vi "Eliminated.vi"(6 "Column":i32, 8 "Row":i32, 9 "Killer":i32, 10 "Team":i32, 11 "AntFarm_MB in":refnum<class "AntFarm_MB.lvclass">) -> (3 "AntFarm_MB out":refnum<class "AntFarm_MB.lvclass">)   [LabVIEW 2017, in "AntFarm_MB.lvclass"]
uses:
  AntFarm_MB.lvclass
  TypeDefs/Cluster_Square Data.ctl
  TypeDefs/ENUM_Position ID.ctl
  Type Defs/Direction Enum.ctl
  Type Defs/Action Enum.ctl
  AntFarm_MB.lvclass/AntFarm_MB.ctl
  Square/Square.lvclass
  Type Defs/SB Type Defs.lvlib
panel:
  out "Data":T1
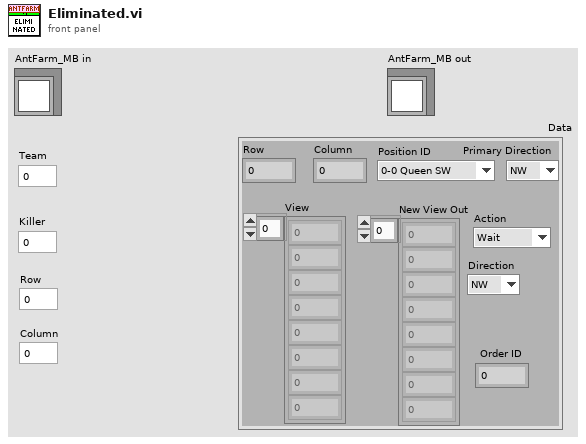
[diagram p1: front panel]
types:
  T1 = typedef "Cluster_Square Data.ctl" = cluster{"Row":i32, "Column":i32, "Position ID":T2, "Primary Direction":T3, "Action":T4, "Direction":T3, "View":i32[], "New View Out":i32[], "Order ID":i32}
  T2 = typedef "ENUM_Position ID.ctl" = enum16{"0-0 Queen SW", "0-1 Path E", "0-2 Queen NW", "0-3 Path W", "1-0 Path S", "1-1 Larva SW", "1-2 Path N", "1-3 Larva NW", "2-0 Queen SE", "2-1 Path W", "2-2 Queen NE", "2-3 Path E", "3-0 Path N", "3-1 Larva SE", "3-2 Path S", "3-3 Larva NE"}
  T3 = typedef "SB Type Defs.lvlib/Direction Enum.ctl" = enum16{"NW", "N", "NE", "E", "SE", "S", "SW", "W"}
  T4 = typedef "SB Type Defs.lvlib/Action Enum.ctl" = enum16{"Wait", "Move", "Attack", "Replicate"}
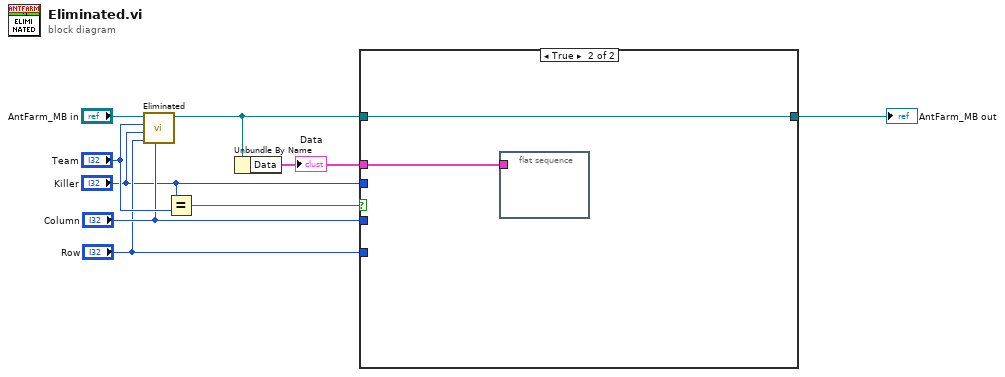
[diagram p0: block diagram]
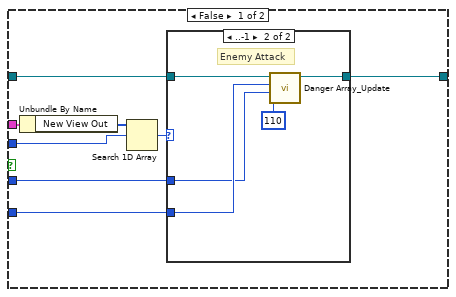
[diagram p2: hidden frame]
diagram:
  n1 = call-parent "Eliminated.vi"("Column"="Column", "Row"="Row", "Killer Index"="Killer", "Team Index"="Team", "Square in"="AntFarm_MB in") -> ("Square out"=w2:refnum<class "AntFarm_MB.lvclass">)  [unwired: 6 in]
  n2 = Equal?(x="Killer", y="Team") -> (x = y?=w6:bool)
  n3 = Unbundle By Name(w2) -> ("Data"=w8:T1)
  "Data" <- w8
  n4 = case shown="True" w6 {
    tunnel: w8 -> [w13 w25]
    tunnel: "Column" -> [w14 _]
    tunnel: "Row" -> [w15 _]
    tunnel: [w16 w24] -> w3
    tunnel: w2 -> [w17 w24]
    tunnel: "Killer" -> [w11 _]
    frame False {
      n5 = Unbundle By Name(w13) -> ("New View Out"=w12:i32[])
      n6 = Search 1D Array(1D array=w12, element=w11) -> (index of element=w10:i32)  [unwired: 1 in]
      n7 = case shown="..-1" w10 {
        tunnel: w17 -> [w18 w23]
        tunnel: [w18 w22] -> w16
        tunnel: w15 -> [_ w21]
        tunnel: w14 -> [_ w20]
        frame 0.. {
        }
        frame ..-1 {
          # "Enemy Attack"
          n8 = call "Danger Array_Update.vi"("Value"=110, "Column"=w20, "Row"=w21, "AntFarm_MB"=w23) -> ("AntFarm_MB Out"=w22:refnum<class "AntFarm_MB.lvclass">)  [unwired: 7 in]
        }
      }
    }
    frame True {
      n9 = flat-sequence {
        tunnel: w25 -> [_]
        frame #0 {
        }
      }
    }
  }
  "AntFarm_MB out" <- w3
